vi "KE622x -- 2182 -A Set Params.vi"(0 "622x Resource In":refnum<visa-resource-name>, 1 "Check For SCPI Errors? (T)":bool=TRUE, 7 "2812 -A Params In":T6={"Auto Range?"=FALSE, "Man / Selected\nRange"=enum."10mV", "Enable Digital\nFilter?"=FALSE, "Filter Type"=enum."Moving", "Filter Count"=10, "Filter\nWindow (%)"=0.01, "Enable Analog\nFilter?"=FALSE, "NPLCs"=5} {"Filter\nWindow (%)" min=0.0 max=10.0 step=0.01 format="%.2f"; "Filter Count" min=1 max=100; "NPLCs" min=1 max=10}, 11 "error in (no error)":errorcluster, 12 "Read Back Set Values? (T)":bool=TRUE) -> (4 "622x Resource Out (dupl)":refnum<visa-resource-name>, 8 "2812 -A Params Out":T6={"Auto Range?"=FALSE, "Man / Selected\nRange"=enum."10mV", "Enable Digital\nFilter?"=FALSE, "Filter Type"=enum."Moving", "Filter Count"=10, "Filter\nWindow (%)"=0.01, "Enable Analog\nFilter?"=FALSE, "NPLCs"=5} {"Filter\nWindow (%)" min=0.0 max=10.0 step=0.01 format="%.2f"; "Filter Count" min=1 max=100; "NPLCs" min=1 max=60}, 15 "error out":errorcluster)   [LabVIEW 2019, in "Keithley 622x.lvlib"]
doc: "Sets the measurement parameters for the 2182/2182A connected to the 622x via the RS232 link."
uses:
  Keithley 622x.lvlib
  Low Level/Typedefs/KE2182 -- Voltage Ranges.ctl
  Low Level/Typedefs/KE2182 -- Filter Type.ctl
  Low Level/Typedefs/KE2182 -- Filter Count.ctl
  Low Level/Typedefs/KE2182 -- Filter Window.ctl
  Low Level/Typedefs/KE2182 -- NPLCs.ctl
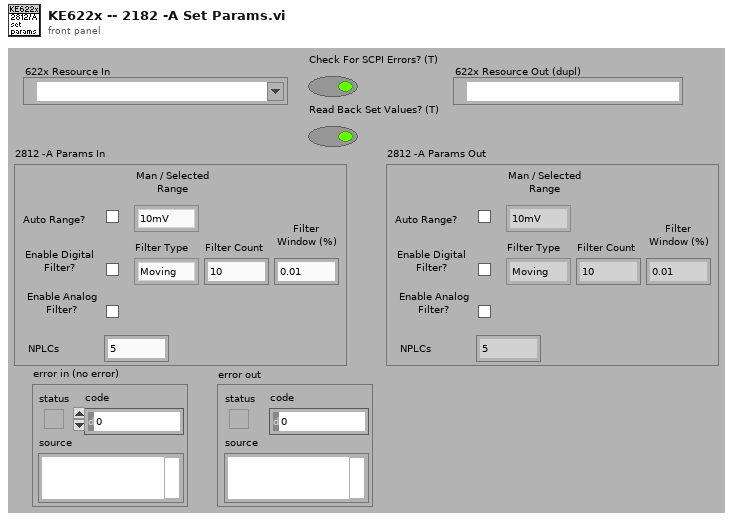
[diagram p1: front panel]
types:
  T1 = typedef "Keithley 622x.lvlib/KE2182 -- Voltage Ranges.ctl" = enum16{"10mV", "100mV", "1V", "10V", "100V"}
  T2 = typedef "Keithley 622x.lvlib/KE2182 -- Filter Type.ctl" = enum16{"Moving", "Repeat"}
  T3 = typedef "Keithley 622x.lvlib/KE2182 -- Filter Count.ctl" = u32
  T4 = typedef "Keithley 622x.lvlib/KE2182 -- Filter Window.ctl" = dbl
  T5 = typedef "Keithley 622x.lvlib/KE2182 -- NPLCs.ctl" = u32
  T6 = cluster{"Auto Range?":bool, "Man / Selected\nRange":T1, "Enable Digital\nFilter?":bool, "Filter Type":T2, "Filter Count":T3, "Filter\nWindow (%)":T4, "Enable Analog\nFilter?":bool, "NPLCs":T5}
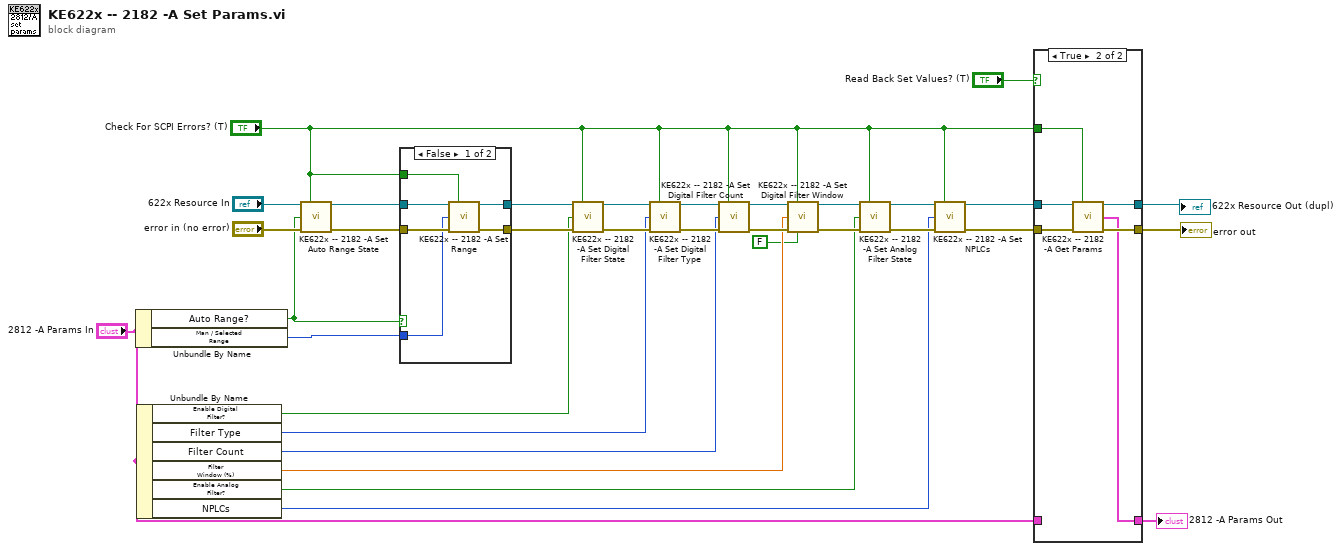
[diagram p0: block diagram]
diagram:
  n1 = Unbundle By Name("2812 -A Params In") -> ("Auto Range?"=w17:bool, "Man / Selected\nRange"=w16:T1)
  n2 = Unbundle By Name("2812 -A Params In") -> ("Enable Digital\nFilter?"=w15:bool, "Filter Type"=w14:T2, "Filter Count"=w13:T3, "Filter\nWindow (%)"=w12:T4, "Enable Analog\nFilter?"=w11:bool, "NPLCs"=w10:T5)
  n3 = call "KE622x -- 2182 -A Set Auto Range State.vi"("622x Resource In"="622x Resource In", "Check For SCPI Errors? (T)"="Check For SCPI Errors? (T)", "Enable Auto Range?"=w17, "error in (no error)"="error in (no error)") -> ("622x Resource Out (dupl)"=w31:refnum<visa-resource-name>, "error out"=w30:errorcluster)  [unwired: 10 in]
  n4 = case shown="False" w17 {
    tunnel: w31 -> [w39 w41]
    tunnel: w30 -> [w38 w40]
    tunnel: [w37 w41] -> w29
    tunnel: [w36 w40] -> w28
    tunnel: w16 -> [w34 _]
    tunnel: "Check For SCPI Errors? (T)" -> [w35 _]
    frame False {
      n5 = call "KE622x -- 2182 -A Set Range.vi"("622x Resource In"=w39, "Check For SCPI Errors? (T)"=w35, "2182/2182A Range"=w34, "error in (no error)"=w38) -> ("622x Resource Out (dupl)"=w37:refnum<visa-resource-name>, "error out"=w36:errorcluster)  [unwired: 10 in]
    }
    frame True {
    }
  }
  n6 = call "KE622x -- 2182 -A Set Digital Filter State.vi"("622x Resource In"=w29, "Check For SCPI Errors? (T)"="Check For SCPI Errors? (T)", "Enable Digital Filter?"=w15, "error in (no error)"=w28) -> ("622x Resource Out (dupl)"=w27:refnum<visa-resource-name>, "error out"=w26:errorcluster)  [unwired: 10 in]
  n7 = call "KE622x -- 2182 -A Set Digital Filter Type.vi"("622x Resource In"=w27, "Check For SCPI Errors? (T)"="Check For SCPI Errors? (T)", "Filter Type"=w14, "error in (no error)"=w26) -> ("622x Resource Out (dupl)"=w25:refnum<visa-resource-name>, "error out"=w24:errorcluster)  [unwired: 10 in]
  n8 = call "KE622x -- 2182 -A Set Digital Filter Count.vi"("622x Resource In"=w25, "Check For SCPI Errors? (T)"="Check For SCPI Errors? (T)", "Filter Count"=w13, "error in (no error)"=w24) -> ("622x Resource Out (dupl)"=w20:refnum<visa-resource-name>, "error out"=w23:errorcluster)  [unwired: 10 in]
  n9 = call "KE622x -- 2182 -A Set Digital Filter Window.vi"("622x Resource In"=w20, "Check For SCPI Errors? (T)"="Check For SCPI Errors? (T)", "Filter Window In (%)"=w12, "error in (no error)"=w23, "Read Back Set Value? (T)"=FALSE) -> ("622x Resource Out (dupl)"=w19:refnum<visa-resource-name>, "error out"=w22:errorcluster)  [unwired: 9 in]
  n10 = call "KE622x -- 2182 -A Set Analog Filter State.vi"("622x Resource In"=w19, "Check For SCPI Errors? (T)"="Check For SCPI Errors? (T)", "Enable Analog Filter?"=w11, "error in (no error)"=w22) -> ("622x Resource Out (dupl)"=w18:refnum<visa-resource-name>, "error out"=w21:errorcluster)  [unwired: 10 in]
  n11 = call "KE622x -- 2182 -A Set NPLCs.vi"("622x Resource In"=w18, "Check For SCPI Errors? (T)"="Check For SCPI Errors? (T)", "2182 -A NPLCs"=w10, "error in (no error)"=w21) -> ("622x Resource Out (dupl)"=w6:refnum<visa-resource-name>, "error out"=w5:errorcluster)  [unwired: 10 in]
  n12 = case shown="True" "Read Back Set Values? (T)" {
    tunnel: "Check For SCPI Errors? (T)" -> [_ w50]
    tunnel: w6 -> [w43 w49]
    tunnel: w5 -> [w42 w48]
    tunnel: "2812 -A Params In" -> [w44 _]
    tunnel: [w44 w45] -> w3
    tunnel: [w43 w47] -> w2
    tunnel: [w42 w46] -> w1
    frame False {
    }
    frame True {
      n13 = call "KE622x -- 2182 -A Get Params.vi"("622x Resource In"=w49, "Check For SCPI Errors? (T)"=w50, "error in (no error)"=w48) -> ("622x Resource Out (dupl)"=w47:refnum<visa-resource-name>, "2812 -A Params"=w45:T6, "error out"=w46:errorcluster)  [unwired: 10 in]
    }
  }
  "622x Resource Out (dupl)" <- w2
  "error out" <- w1
  "2812 -A Params Out" <- w3
